vi "ApplyPropertyTemplateToMethod.vi"(0 "ClassWriterGOOP300 in":refnum<class "ClassWriterGOOP400.lvclass">, 1 "VIRef":refnum<vi>, 2 "ClassRef":refnum<vi>, 3 "PropertyName":string, 4 "MethodTemplateName":string, 5 "error in (no error)":errorcluster) -> (14 "ClassWriterGOOP300 out":refnum<class "ClassWriterGOOP400.lvclass">, 19 "error out":errorcluster)   [LabVIEW 2020, in "ClassWriterGOOP400.lvclass"]
uses:
  <resource>/Framework/Providers/Open_GDS/ClassProviders/Provider_EndevoGOOP400/ClassWriterGOOP400_class/ClassWriterGOOP400.lvclass
  <resource>/Framework/Providers/Open_GDS/ClassProviders/Provider_LvNativeClass/ClassWriterNative_class/ClassWriterNative.lvclass
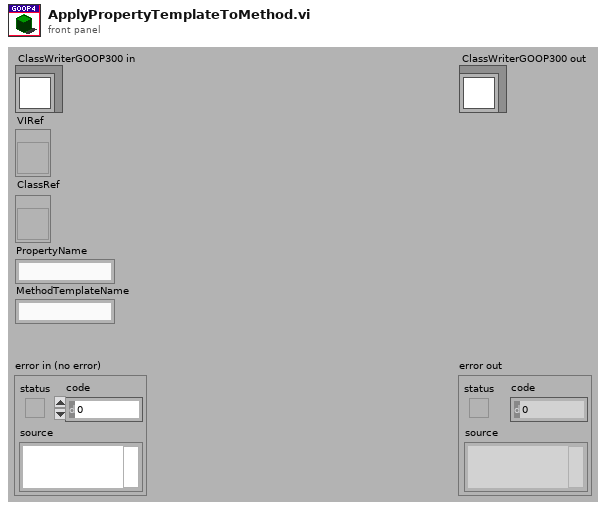
[diagram p1: front panel]
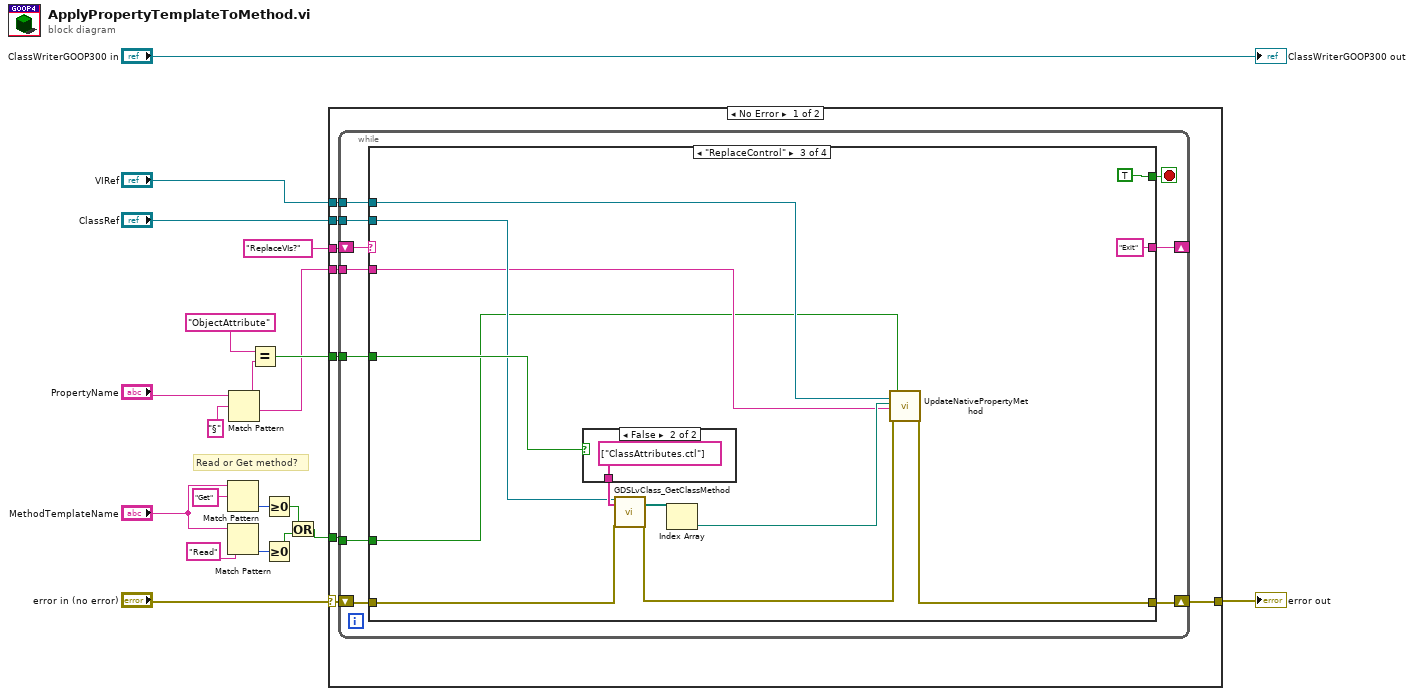
[diagram p0: block diagram]
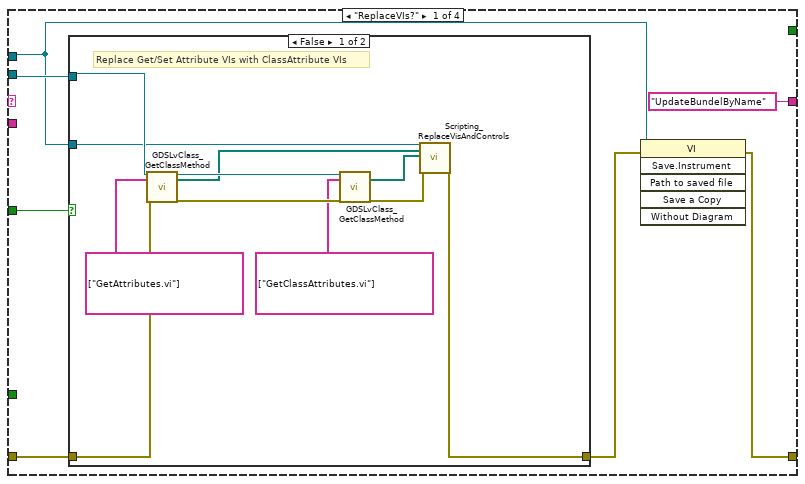
[diagram p2: hidden frame]
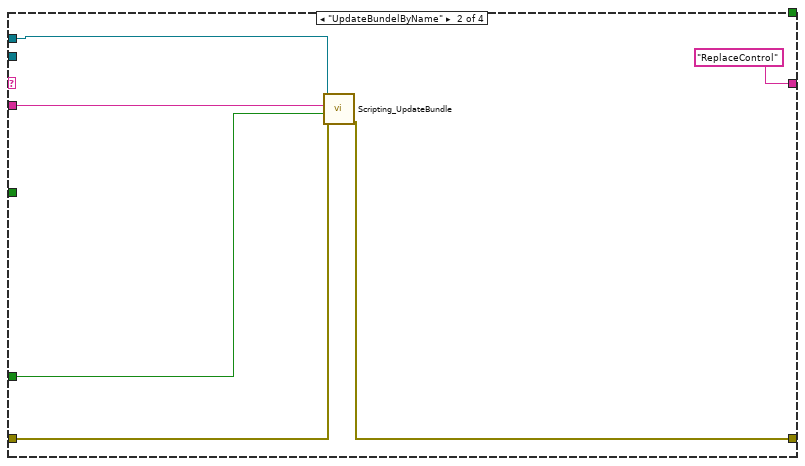
[diagram p4: hidden frame]
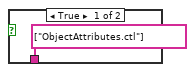
[diagram p5: hidden frame]
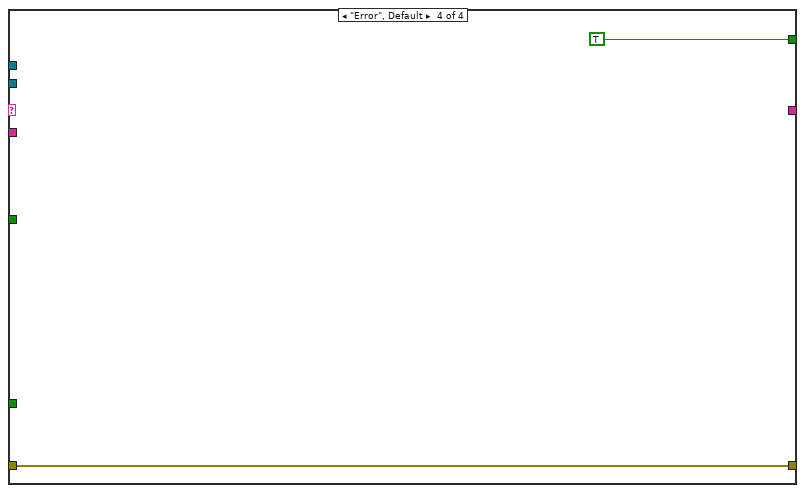
[diagram p6: hidden frame]
diagram:
  # "Read or Get method?"
  n1 = Match Pattern(string="MethodTemplateName", regular expression="Get") -> (offset past match=w5:i32)  [unwired: 1 in, 3 out]
  n2 = Match Pattern(string="MethodTemplateName", regular expression="Read") -> (offset past match=w7:i32)  [unwired: 1 in, 3 out]
  n3 = Match Pattern(string="PropertyName", regular expression="§" ("search string")) -> (before substring=w18:string, after substring=w15:string)  [unwired: 1 in, 2 out]
  n4 = Equal?(x="ObjectAttribute" ("string"), y=w18) -> (x = y?=w16:bool)
  n5 = Greater Or Equal To 0?(x=w5) -> (x >= 0?=w3:bool)
  n6 = Greater Or Equal To 0?(x=w7) -> (x >= 0?=w4:bool)
  n7 = Or(x=w3, y=w4) -> (x .or. y?=w1:bool)
  n8 = case shown="No Error" "error in (no error)" {
    selector: "error in (no error)" -> [w22 w81]
    tunnel: "ReplaceVIs?" -> [w28 _]
    tunnel: "VIRef" -> [w27 _]
    tunnel: "ClassRef" -> [w26 _]
    tunnel: w1 -> [w25 _]
    tunnel: w15 -> [w24 _]
    tunnel: [w23 w81] -> w9
    tunnel: w16 -> [w21 _]
    frame No Error {
      n9 = while {
        tunnel: w27 -> [w38]
        tunnel: w24 -> [w37]
        shift-right: [w35] -> w23
        shift-left: w22 -> [w36]
        shift-right: [w33] -> _
        shift-left: w28 -> [w34]
        tunnel: w26 -> [w31]
        tunnel: w25 -> [w30]
        tunnel: w21 -> [w29]
        stop <- w32 stop-if-true
        n10 = case shown="\"ReplaceControl\"" w34 {
          tunnel: w38 -> [w40 w62 w65 _]
          tunnel: w37 -> [_ w59 w66 _]
          tunnel: w36 -> [w43 w61 w68 w79]
          tunnel: [w41 w60 w67 w79] -> w35
          tunnel: ["UpdateBundelByName" "ReplaceControl" "Exit" _] -> w33
          tunnel: [_ _ TRUE TRUE] -> w32
          tunnel: w31 -> [w44 _ w70 _]
          tunnel: w30 -> [_ w58 w64 _]
          tunnel: w29 -> [w39 _ w71 _]
          frame "ReplaceVIs?" {
            n11 = case shown="False" w39 {
              tunnel: w44 -> [w54 _]
              tunnel: w40 -> [w46 _]
              tunnel: w43 -> [w53 w57]
              tunnel: [w56 w57] -> w42
              frame False {
                # "Replace Get/Set Attribute VIs with ClassAttribute VIs"
                n12 = call <resource>:"GDSLvClass_GetClassMethod.vi"("Class Refnum In"=w54, "VINames"=string[] ["GetAttributes.vi"], "error in (no error)"=w53) -> ("Class Refnum Out"=w52:refnum<vi>, "ViPaths"=w48:path[], "error out"=w51:errorcluster)  [unwired: 13 in, 1 out]
                n13 = call <resource>:"GDSLvClass_GetClassMethod.vi"("Class Refnum In"=w52, "VINames"=string[] ["GetClassAttributes.vi"], "error in (no error)"=w51) -> ("ViPaths"=w47:path[], "error out"=w50:errorcluster)  [unwired: 13 in, 2 out]
                n14 = call <resource>:"Scripting_ReplaceVisAndControls.vi"("ViRef"=w46, "OldVIsAndControls"=w48, "NewVIsAndControls"=w47, "error in (no error)"=w50) -> ("error out"=w56:errorcluster)  [unwired: 14 in, 1 out]
              }
              frame True {
              }
            }
            n15 = invoke class="VI" method="Save.Instrument"(reference=w40, error in=w42) -> (error out=w41:errorcluster)  [unwired: 4 in, 5 out]
          }
          frame "UpdateBundelByName" {
            n16 = call <resource>:"Scripting_UpdateBundle.vi"("error in (no error)"=w61, "Boolean"=w58, "PropertyName"=w59, "VI in"=w62) -> ("error out"=w60:errorcluster)  [unwired: 7 in]
          }
          frame "ReplaceControl" {
            n17 = case shown="False" w71 {
              tunnel: [string[] ["ObjectAttributes.ctl"] ("VINames") string[] ["ClassAttributes.ctl"] ("VINames")] -> w73
              frame True {
              }
              frame False {
              }
            }
            n18 = call <resource>:"GDSLvClass_GetClassMethod.vi"("Class Refnum In"=w70, "VINames"=w73, "error in (no error)"=w68) -> ("ViPaths"=w74:path[], "error out"=w69:errorcluster)  [unwired: 13 in, 2 out]
            n19 = Index Array(array=w74) -> (element=w72:path)  [unwired: 1 in]
            n20 = call <resource>:"UpdateNativePropertyMethod.vi"("VI"=w65, "TypeDefControl"=w72, "Property"=w66, "error IO"=w69, "GetMethod"=w64) -> ("error out"=w67:errorcluster)  [unwired: 14 in]
          }
          frame "Error", Default {
          }
        }
      }
    }
    frame Error {
    }
  }
  "error out" <- w9
  "ClassWriterGOOP300 out" <- "ClassWriterGOOP300 in"
